vi "Parse Response Message.vi"(8 "error in":errorcluster, 11 "Thorlabs In":refnum<class "Thorlabs.lvclass">) -> (0 "error out":errorcluster, 3 "Thorlabs Out":refnum<class "Thorlabs.lvclass">)   [LabVIEW 2018, in "Thorlabs.lvlib" / "Thorlabs.lvclass"]
doc: "There is no respone message, so instead we query the status here so it's up to date.\n\nCreator: Slade Jeppesen\nCreated Date: 09/29/20"
uses:
  Thorlabs.lvclass
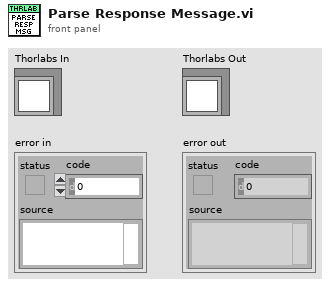
[diagram p1: front panel]
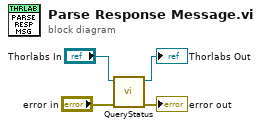
[diagram p0: block diagram]
diagram:
  n1 = call "QueryStatus.vi"("Error In"="error in", "Thorlabs In"="Thorlabs In") -> ("Error Out"=→"error out":errorcluster, "Thorlabs Out"=→"Thorlabs Out":refnum<class "Thorlabs.lvclass">)  [unwired: 8 in]
